vi "AR-Highlight-execution.vi"(6 "Current row":i32, 7 "Action":enum16{"Init", "Highlight"}(ring), 8 "error in":errorcluster, 10 "Table Ref":refnum<vi>, 11 "file (use dialog)":path) -> (0 "error out":errorcluster, 3 "Commands":T1[](array[typedef]))   [LabVIEW 2021]
uses:
  Controls/Command_cluster.ctl
  Controls/Command_Enum.ctl
panel:
  in  "Table":string[][](table)
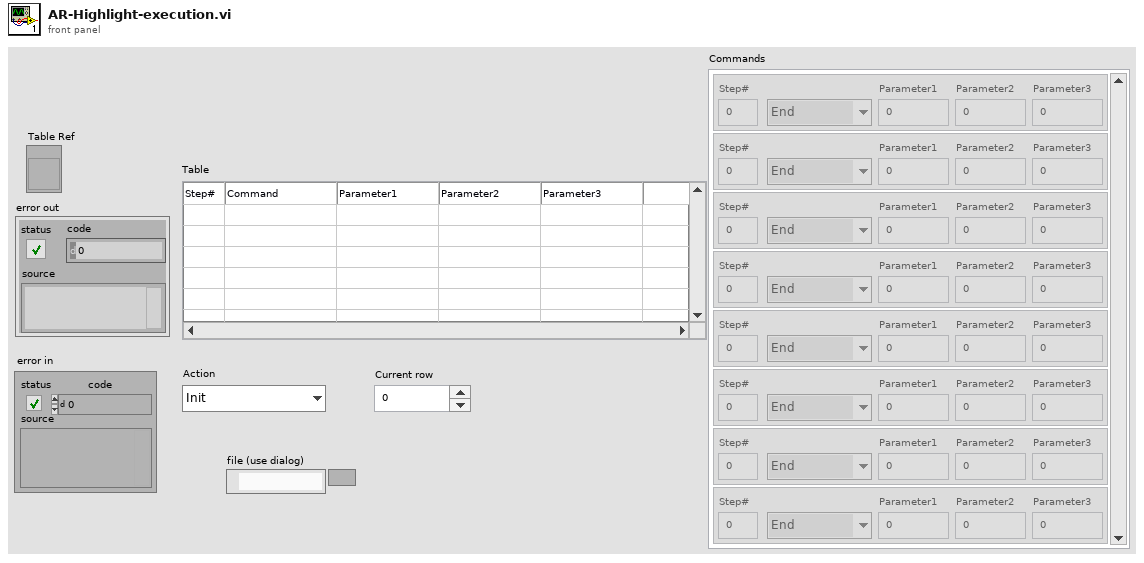
[diagram p1: front panel]
types:
  T1 = typedef "Command_cluster.ctl" = cluster{"Step#":dbl, "Commands":T2, "Parameter1":dbl, "Parameter2":dbl, "Parameter3":dbl}
  T2 = typedef "Command_Enum.ctl" = enum16{"End", "Home All", "X Home", "Y Home", "X Move Rel", "X Move Abs", "Y Move Rel", "Y Move Abs", "Wait", "Repeat", "Reset Intlk Timer", "Laser Sys ON", "Laser ENA"}
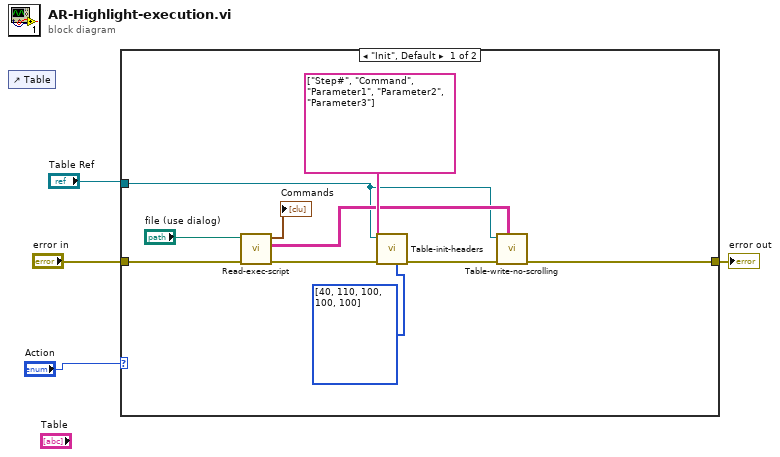
[diagram p0: block diagram]
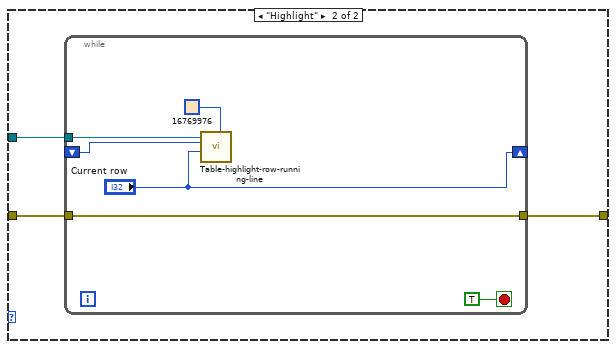
[diagram p2: hidden frame]
diagram:
  n1 = control-ref of="Table"() -> ()  [unwired: 1 out]
  n2 = case shown="\"Init\", Default" "Action" {
    tunnel: "Table Ref" -> [w9 w17]
    tunnel: "error in" -> [w6 w16]
    tunnel: [w5 w15] -> w2
    frame "Init", Default {
      n3 = call "Read-exec-script.vi"("error in"=w6, "file (use dialog)"="file (use dialog)") -> ("error out"=w13:errorcluster, "Commands Str Array"=w10:string[][], "Commands"=→"Commands":T1[])  [unwired: 7 in]
      n4 = call "Table-init-headers.vi"("Col Widths"=u32[] [40, 110, 100, 100, 100], "Col Names"=string[] ["Step#", "Command", "Parameter1", "Parameter2", "Parameter3"], "error in"=w13, "Table in"=w9) -> ("error out"=w8:errorcluster)  [unwired: 7 in]
      n5 = call "Table-write-no-scrolling.vi"("Table Data In"=w10, "error in"=w8, "Table in"=w9) -> ("error out"=w5:errorcluster)  [unwired: 8 in]
    }
    frame "Highlight" {
      n6 = while {
        tunnel: w17 -> [w23]
        tunnel: w16 -> [w21]
        tunnel: [w21] -> w15
        shift-right: ["Current row"] -> _
        shift-left: _ -> [w18]
        stop <- TRUE stop-if-true
        n7 = call "Table-highlight-row-running-line.vi"("Highlight"=u32 16769976, "Current row"="Current row", "Last row"=w18, "Table in"=w23) -> ()  [unwired: 8 in]
      }
    }
  }
  "error out" <- w2
